vi "PRUEBA_FPGA_8a_2ws_BIdireccional.vi"() -> ()   [LabVIEW 2015]
doc: "This VI reads a buffer of single point values from all four channels of the NI 923x and places the acquired data into a DMA FIFO."
uses:
  <vilib>/LabVIEW Targets/FPGA/cRIO/shared/nicrio_ModuleControls/nicrio_cRIO-9234_DataRatesRing2.ctl
  <vilib>/LabVIEW Targets/FPGA/cRIO/shared/nicrio_ModuleControls/nicrio_BasicConversionTime.ctl
  <vilib>/rvi/Emulation/niFpgaGetClockAttributes.vi
  <vilib>/rvi/Emulation/niFpgaSctlEmulationGetInTimedLoop.vi
  <vilib>/rvi/Emulation/niFpgaEmulationReportErrorSimple.vi
  <vilib>/rvi/eio/common/nirviEmuTemplateMethod_errors.vi
  <vilib>/rvi/Emulation/niFpgaCriticalErrorInLSC.vi
  <vilib>/rvi/eio/common/nirviEmuTemplatePropertySet_errors.vi
  <vilib>/rvi/Emulation/niFpgaProcessEmulError.vi
  <vilib>/rvi/interface/RandomDataEmulation/niFpgaRandomDataHandleErrors.vi
  <vilib>/eio/EIONode/EIONode.xnode
  <vilib>/eio/EIOPropertyNode/EIOPropertyNode.xnode
  <vilib>/rvi/DataTransferAndStorage/Container/XNode/niFpgaContainer.xnode
  <vilib>/rvi/interface/RandomDataEmulation/nirviRandomDataFpgaReadWriteTemplate.vi
  <vilib>/rvi/eio/common/nirviEmuTemplatePropertyGet_errors.vi
  <vilib>/rvi/eio/common/nirviEmuTemplatePropertyGet_noerrors.vi
  <vilib>/rvi/eio/common/nirviEmuTemplatePropertySet_noerrors.vi
panel:
  out "appended array":fxp<+/-,24,4>[](array[numeric])
  in  "Cycles to Filter":u16=5
  in  "Offset_WS2":fxp<+/-,24,-4>=0.000999998301267624 format="%.27g"
  in  "Canal cero WS2?":bool=TRUE
  out "NºRuedas 2":i32
  out "Nº Ruedas 1":i32
  out "Parar":bool
  out "RuedaDetectada2?":bool
  out "RuedaDetectada1?":bool
  out "Rueda2?":i16
  out "WhlCnt2":fxp<+/-,24,-4> format="%.27g"
  in  "Digital?":bool=TRUE
  out "Numeric 2":i32
  out "WhlCnt1":fxp<+/-,24,-4> format="%.27g"
  in  "Offset_WS1":fxp<+/-,24,-4>=0.000999998301267624 format="%.27g"
  out "Rueda1?":i16
  in  "Conversion Time":T1
  in  "Canal cero WS1?":bool=TRUE
  in  "Count(mSec)":u32=2
  out "Chassis Temperature":i16
  out "Detector de\npresencia":bool
  in  "Fotocélula":bool
  out "DC OK":bool
  in  "Data Rate":T2=2 items=["51.200 kS/s (NI 9234)"=1, "25.600 kS/s (NI 9234)"=2, "17.067 kS/s (NI 9234)"=3, "12.800 kS/s (NI 9234)"=4, "10.240 kS/s (NI 9234)"=5, "8.533 kS/s (NI 9234)"=6, "7.314 kS/s (NI 9234)"=7, "6.400 kS/s (NI 9234)"=8, "5.689 kS/s (NI 9234)"=9, "5.120 kS/s (NI 9234)"=10, "4.654 kS/s (NI 9234)"=11, "4.267 kS/s (NI 9234)"=12, "3.938 kS/s (NI 9234)"=13, "3.657 kS/s (NI 9234)"=14, "3.413 kS/s (NI 9234)"=15, "3.200 kS/s (NI 9234)"=16, "3.012 kS/s (NI 9234)"=17, "2.845 kS/s (NI 9234)"=18, "2.695 kS/s (NI 9234)"=19, "2.560 kS/s (NI 9234)"=20, "2.438 kS/s (NI 9234)"=21, "2.328 kS/s (NI 9234)"=22, "2.226 kS/s (NI 9234)"=23, "2.133 kS/s (NI 9234)"=24, "2.048 kS/s (NI 9234)"=25, "1.969 kS/s (NI 9234)"=26, "1.896 kS/s (NI 9234)"=27, "1.829 kS/s (NI 9234)"=28, "1.765 kS/s (NI 9234)"=29, "1.707 kS/s (NI 9234)"=30, "1.652 kS/s (NI 9234)"=31]
  out "Buffer Overflow":bool
  in  "Stop":bool
  out "Buffer Underflow":bool
  out "Error Out":errorcluster
  # "For instructions, and select Help>>Show Context Help and hover over the icon."
  # "Timing Parameters"
  # "Output Parameters"
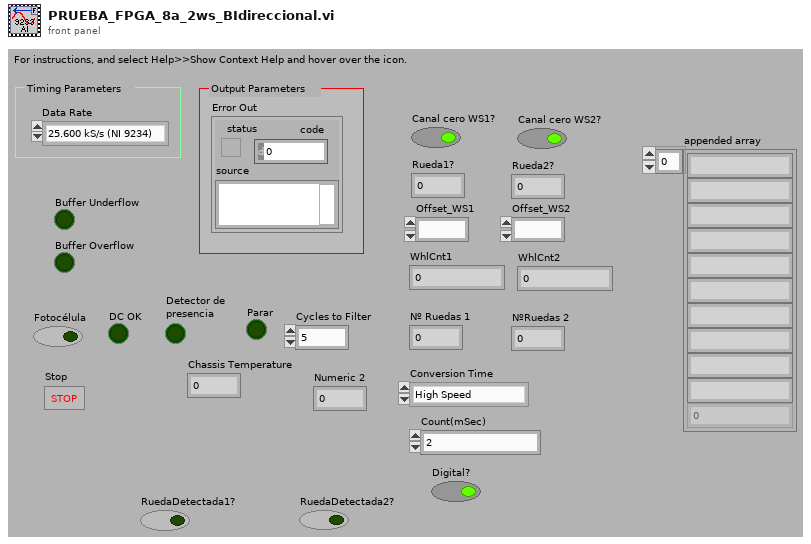
[diagram p1: front panel]
types:
  T1 = typedef "nicrio_BasicConversionTime.ctl" = enum8{"High Speed", "High Resolution"}
  T2 = typedef "nicrio_cRIO-9234_DataRatesRing2.ctl" = u8
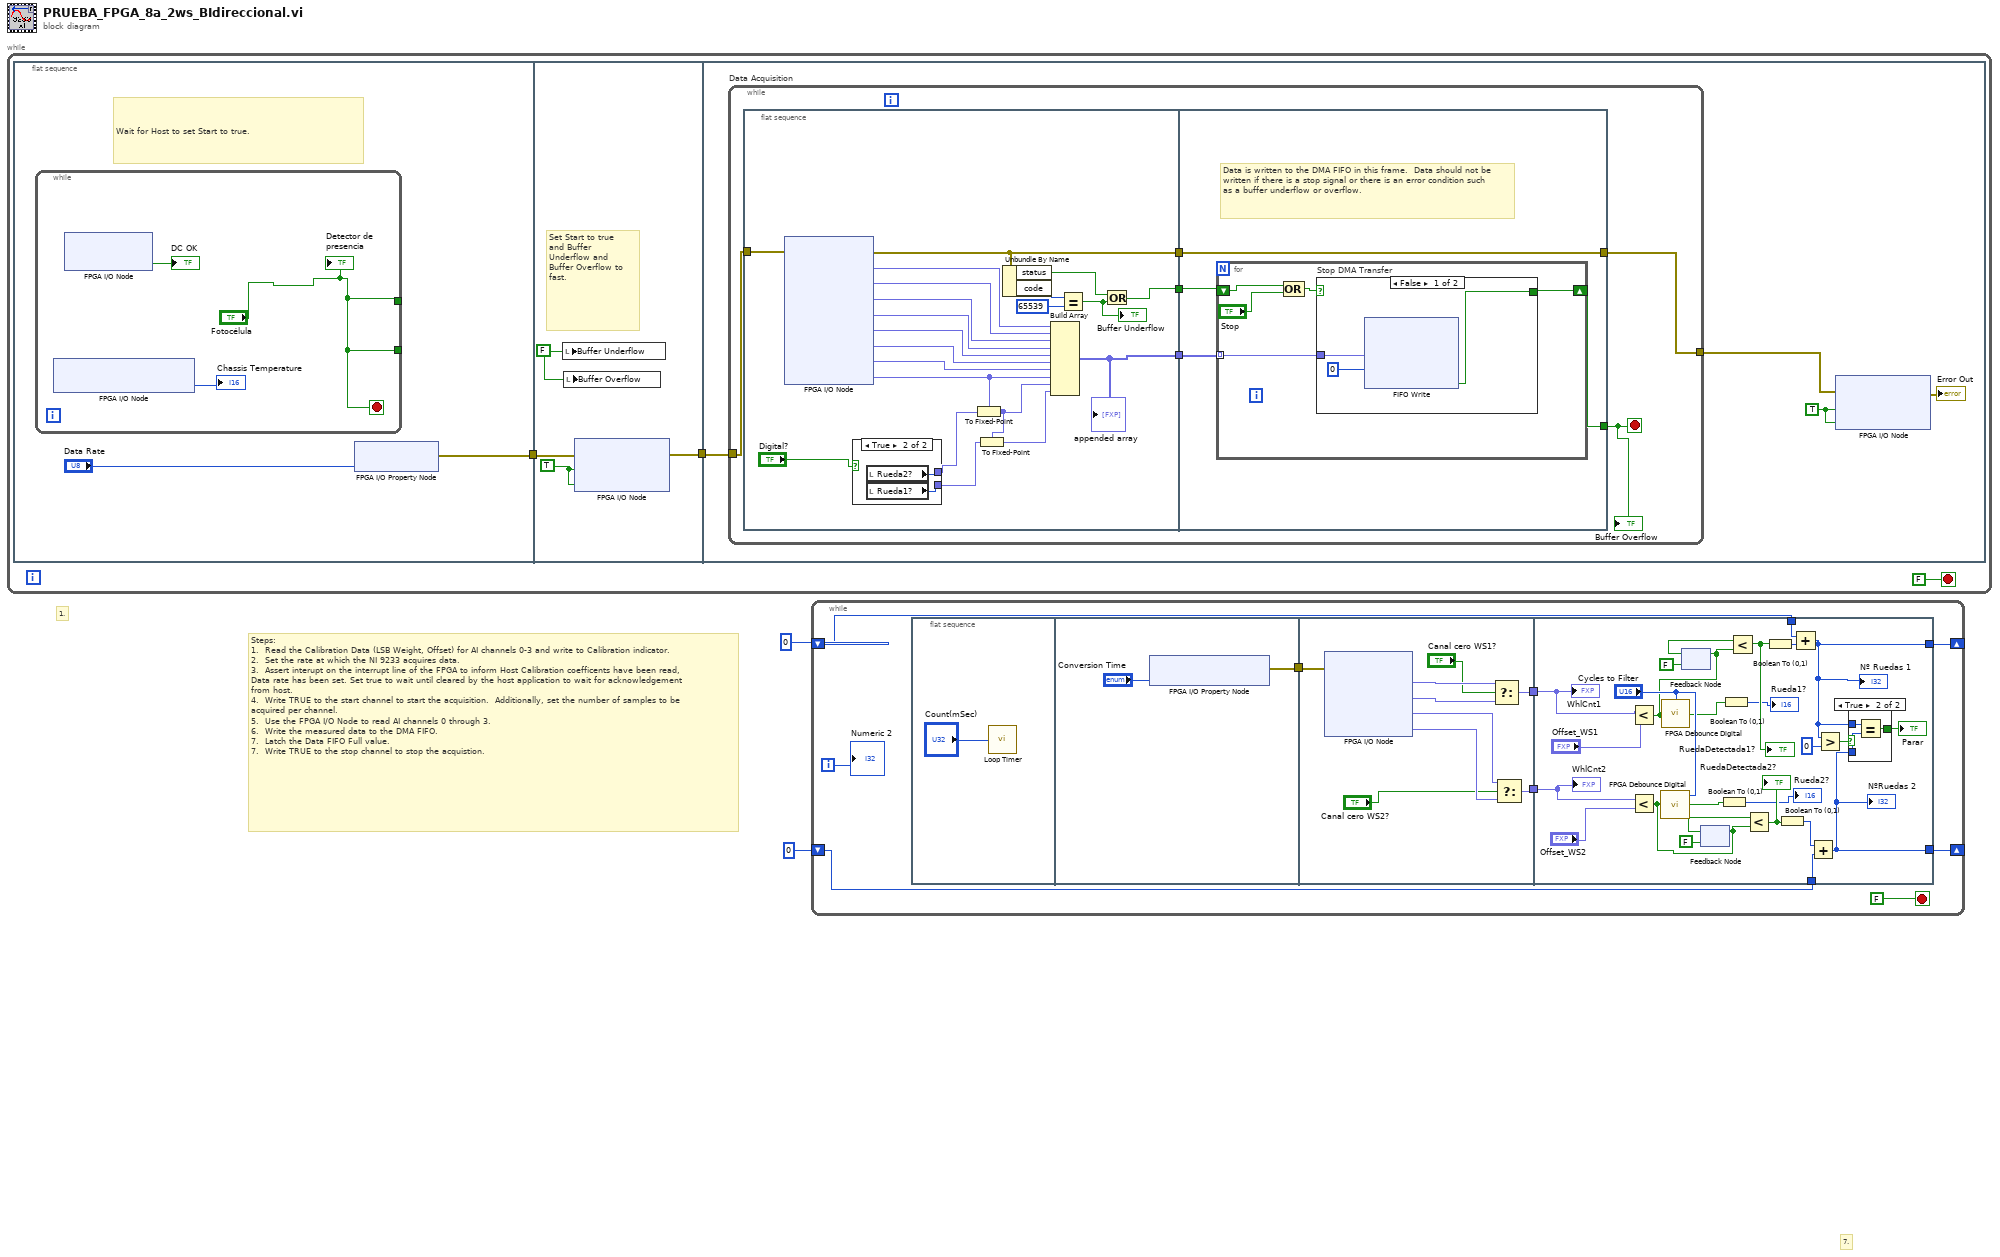
[diagram p0: block diagram]
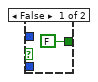
[diagram p2: hidden frame]
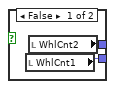
[diagram p3: hidden frame]
diagram:
  # "Steps: \n1.  Read the Calibration Data (LSB Weight, Offset) for AI channels 0-3 and write to Calibration indicator.\n2.  Set the rate at which the NI 9233 acquires data. \n3.  Assert interupt on the interrupt line of the FPGA to inform Host Calibration coefficents have been read, Data rate has been set. Set true to wait until cleared by the host application to wait for acknowledgement from host.\n4.  Write TRUE to the start channel to start the acquisition.  Additionally, set the number of samples to be acquired per channel.\n5.  Use the FPGA I/O Node to read AI channels 0 through 3. \n6.  Write the measured data to the DMA FIFO.\n7.  Latch the Data FIFO Full value.\n7.  Write TRUE to the stop channel to stop the acquistion."
  # "1."
  # "7."
  n1 = while {
    stop <- FALSE stop-if-true
    n2 = flat-sequence "MainSeq" {
      tunnel: [w7] -> w4
      tunnel: w4 -> [w13]
      tunnel: [w12] -> w3
      tunnel: w3 -> [w18]
      frame #0 {
        # "Wait for Host to set Start to true."
        n3 = while "initWait" {
          tunnel: ["Fotocélula"] -> _
          tunnel: ["Fotocélula"] -> _
          stop <- "Fotocélula" stop-if-true
          n4 = xnode "FPGA I/O Node"() -> ("Chassis Temperature"=→"Chassis Temperature":i16)  [unwired: 1 in, 1 out]
          n5 = xnode "FPGA I/O Node"() -> ("Mod3/DI2"=→"DC OK":bool)  [unwired: 2 in, 2 out]
          "Detector de\npresencia" <- "Fotocélula"
        }
        n6 = xnode "FPGA I/O Property Node"("Data Rate"="Data Rate") -> ("error out"=w7:errorcluster)  [unwired: 2 in, 1 out]
      }
      frame #1 {
        w11 = TRUE
        w14 = FALSE ("Late? (Latched)")
        # "Set Start to true and Buffer Underflow and Buffer Overflow to fast."
        n7 = local write "Buffer Underflow"(w14) -> ()
        n8 = local write "Buffer Overflow"(w14) -> ()
        n9 = xnode "FPGA I/O Node"("error in"=w13, "Mod1/Start"=w11, "Mod2/Start"=w11) -> ("error out"=w12:errorcluster)  [unwired: 2 in, 2 out]
      }
      frame #2 {
        w15 = TRUE
        n10 = while "Data Acquisition" {
          tunnel: w18 -> [w22]
          tunnel: [w21] -> w16
          stop <- w19 stop-if-true
          n11 = flat-sequence "Data Acquisition Sequence" {
            tunnel: [w44] -> w24
            tunnel: [w35] -> w23
            tunnel: w22 -> [w43]
            tunnel: [w42] -> w20
            tunnel: w24 -> [w53]
            tunnel: w23 -> [w52]
            tunnel: [w51] -> w19
            tunnel: [w50] -> w21
            tunnel: w20 -> [w50]
            frame #0 {
              n12 = xnode "FPGA I/O Node"("error in"=w43) -> ("error out"=w42:errorcluster, "Mod1/AI0"=w45:fxp<+/-,24,4>, "Mod1/AI1"=w38:fxp<+/-,24,4>, "Mod1/AI2"=w37:fxp<+/-,24,4>, "Mod1/AI3"=w36:fxp<+/-,24,4>, "Mod2/AI0"=w33:fxp<+/-,24,4>, "Mod2/AI1"=w32:fxp<+/-,24,4>, "Mod2/AI2"=w31:fxp<+/-,24,4>, "Mod2/AI3"=w30:fxp<+/-,24,4>)  [unwired: 8 in, 8 out]
              n13 = case shown="True" "Digital?" {
                tunnel: [w47 w49] -> w29
                tunnel: [w46 w48] -> w27
                frame False {
                  n14 = local read "WhlCnt1"() -> (w46:fxp<+/-,24,-4>)
                  n15 = local read "WhlCnt2"() -> (w47:fxp<+/-,24,-4>)
                }
                frame True {
                  n16 = local read "Rueda2?"() -> (w49:i16)
                  n17 = local read "Rueda1?"() -> (w48:i16)
                }
              }
              n18 = To Fixed-Point(fixed-point type=w30, number=w29) -> (fixed-point=w26:fxp<+/-,24,4>)
              n19 = To Fixed-Point(fixed-point type=w26, number=w27) -> (fixed-point=w25:fxp<+/-,24,4>)
              n20 = Unbundle By Name(w42) -> ("status"=w34:bool, "code"=w41:i32)
              n21 = Build Array(w45, w38, w37, w36, w33, w32, w31, w30, w26, w25) -> (w44:fxp<+/-,24,4>[])
              "appended array" <- w44
              n22 = Equal?(x=w41, y=65539) -> (x = y?=w39:bool)
              "Buffer Underflow" <- w39
              n23 = Or(x=w34, y=w39) -> (x .or. y?=w35:bool)
            }
            frame #1 {
              # "Data is written to the DMA FIFO in this frame.  Data should not be written if there is a stop signal or there is an error condition such as a buffer underflow or overflow."
              n24 = for "DMAWriteLoop" {
                tunnel: w53 -> [w58] mode=indexing
                shift-right: [w57] -> w51
                shift-left: w52 -> [w56]
                n25 = Compound Arithmetic op=OR(w56, "Stop") -> (w55:bool)
                n26 = case "Stop DMA Transfer" shown="False" w55 {
                  selector: w55 -> [_ w62]
                  tunnel: w58 -> [w59 _]
                  tunnel: [w61 w62] -> w57
                  frame False {
                    n27 = xnode ("FIFO Write")("Element"=w59, "Timeout"=0) -> ("Timed Out?"=w61:bool)  [unwired: 1 in, 1 out]
                  }
                  frame True {
                  }
                }
              }
            }
          }
          "Buffer Overflow" <- w19
        }
        n28 = xnode "FPGA I/O Node"("error in"=w16, "Mod1/Stop"=w15, "Mod2/Stop"=w15) -> ("error out"=→"Error Out":errorcluster)  [unwired: 2 in, 2 out]
      }
    }
  }
  n29 = while {
    shift-right: [w68] -> _
    shift-left: 0 -> [w67]
    shift-right: [w65] -> _
    shift-left: 0 -> [w66]
    i -> [w64]
    stop <- FALSE stop-if-true
    n30 = flat-sequence {
      tunnel: [w73] -> w70
      tunnel: [w83] -> w71
      tunnel: w70 -> [w77]
      tunnel: [w80] -> w69
      tunnel: w71 -> [w109]
      tunnel: w69 -> [w107]
      tunnel: [w97] -> w68
      tunnel: w67 -> [w104]
      tunnel: w66 -> [w102]
      tunnel: [w96] -> w65
      frame #0 {
        n31 = call "Loop Timer"("Count(mSec)"="Count(mSec)") -> ()  [unwired: 1 out]
      }
      frame #1 {
        n32 = xnode "FPGA I/O Property Node"("Conversion Time"="Conversion Time") -> ("error out"=w73:errorcluster)  [unwired: 2 in, 1 out]
      }
      frame #2 {
        n33 = xnode "FPGA I/O Node"("error in"=w77) -> ("Mod4/AI0"=w82:fxp<+/-,24,-4>, "Mod4/AI1"=w81:fxp<+/-,24,-4>, "Mod4/AI2"=w79:fxp<+/-,24,-4>, "Mod4/AI3"=w78:fxp<+/-,24,-4>)  [unwired: 4 in, 5 out]
        n34 = Select(t=w82, s="Canal cero WS1?", f=w81) -> (s? t:f=w83:fxp<+/-,24,-4>)
        n35 = Select(t=w79, s="Canal cero WS2?", f=w78) -> (s? t:f=w80:fxp<+/-,24,-4>)
      }
      frame #3 {
        n36 = Less?(x=w109, y="Offset_WS1") -> (x < y?=w87:bool)
        n37 = Less?(x=w107, y="Offset_WS2") -> (x < y?=w85:bool)
        n38 = call "FPGA Debounce Digital.vi"("Input Signal"=w85, "Cycles to Filter"="Cycles to Filter") -> ("Output Filtered Signal"=w84:bool)
        n39 = call "FPGA Debounce Digital.vi"("Input Signal"=w87, "Cycles to Filter"="Cycles to Filter") -> ("Output Filtered Signal"=w86:bool)
        n40 = feedback-in #1(w87) -> ()
        n41 = feedback #1(FALSE) -> (w105:bool)
        n42 = feedback #2(FALSE) -> (w98:bool)
        n43 = feedback-in #2(w85) -> ()
        n44 = Boolean To (0,1)(Boolean=w84) -> (0, 1=→"Rueda2?":i16)
        n45 = Boolean To (0,1)(Boolean=w86) -> (0, 1=→"Rueda1?":i16)
        n46 = Less?(x=w105, y=w87) -> (x < y?=w93:bool)
        "RuedaDetectada1?" <- w93
        n47 = Less?(x=w98, y=w85) -> (x < y?=w92:bool)
        "RuedaDetectada2?" <- w92
        n48 = Boolean To (0,1)(Boolean=w93) -> (0, 1=w89:i16)
        n49 = Boolean To (0,1)(Boolean=w92) -> (0, 1=w94:i16)
        n50 = Add(x=w104, y=w89) -> (x+y=w97:i32)
        "Nº Ruedas 1" <- w97
        n51 = Add(x=w94, y=w102) -> (x+y=w96:i32)
        "NºRuedas 2" <- w96
        n52 = Greater?(x=w97, y=i64 0) -> (0:w99:bool)
        n53 = case shown="True" w99 {
          tunnel: w96 -> [_ w113]
          tunnel: w97 -> [_ w112]
          tunnel: [FALSE w111] -> w101
          frame False {
          }
          frame True {
            n54 = Equal?(x=w112, y=w113) -> (x = y?=w111:bool)
          }
        }
        "Parar" <- w101
        "WhlCnt1" <- w109
        "WhlCnt2" <- w107
      }
    }
    "Numeric 2" <- w64
  }
